vi "PID_TempControl.vi"() -> ()   [LabVIEW 2021]
uses:
  <vilib>/addons/control/pid/pid.llb/PID (DBL).vi
  <vilib>/addons/control/pid/NI_PID_pid.lvlib
panel:
  out "Meter":dbl(knob) scale=0.0..100.0
  in  "Dial":dbl(knob) scale=0.0..150.0
  in  "stop":bool
  out "Grafico de salidas":T1(graph)
  in  "PID gains":T2={"proportional gain (Kc)"=1.0, "integral time (Ti, min)"=0.01, "derivative time (Td, min)"=0.0} {"derivative time (Td, min)" format="%.3f"; "integral time (Ti, min)" format="%.3f"; "proportional gain (Kc)" format="%.3f"}
  out "Termometro":dbl(slide) scale=-2.0..150.0
  in  "Seleccionar temperatura (°c)":dbl(knob) scale=-2.0..150.0
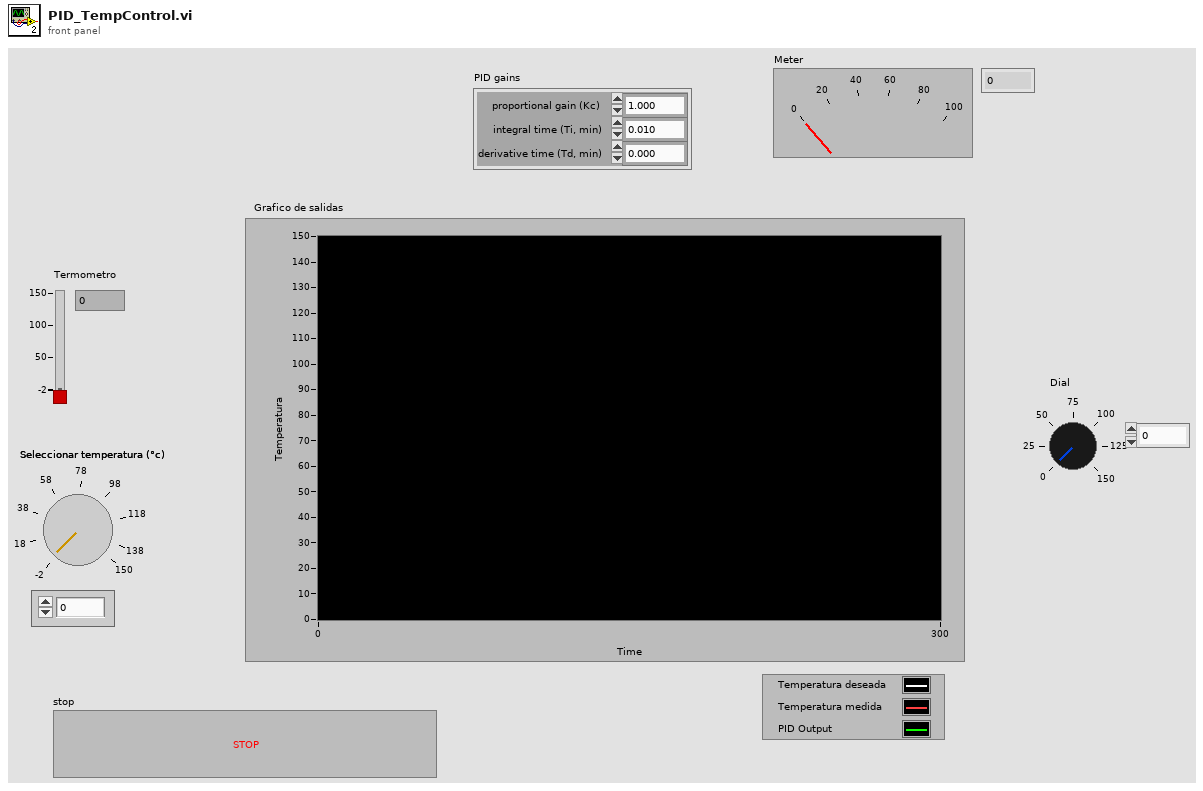
[diagram p1: front panel]
types:
  T1 = cluster{"Seleccionar temperatura (°c)":dbl, dbl, "output":dbl}
  T2 = cluster{"proportional gain (Kc)":dbl, "integral time (Ti, min)":dbl, "derivative time (Td, min)":dbl}
  T3 = cluster{"Seleccionar temperatura (°c)":dbl, "Dial":dbl, "output":dbl}
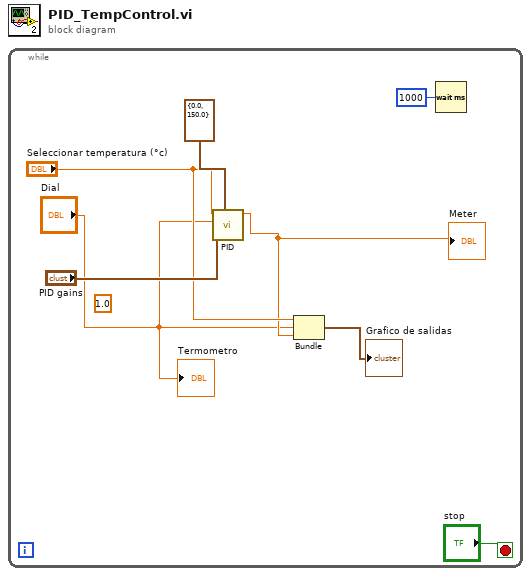
[diagram p0: block diagram]
diagram:
  n1 = while {
    stop <- "stop" stop-if-true
    (unwired) 1.0 ("y")
    n2 = call-poly <vilib>:"PID.vi"("output range"=cluster{"output low":dbl, "output high":dbl} {"output low"=0.0, "output high"=150.0}, "PID gains"="PID gains", "process variable"="Dial", "setpoint"="Seleccionar temperatura (°c)") -> ("output"=w2:dbl)  [unwired: 6 in, 1 out]
    "Meter" <- w2
    n3 = Bundle("Seleccionar temperatura (°c)"="Seleccionar temperatura (°c)", "Dial"="Dial", "output"=w2) -> (→"Grafico de salidas":T3)  [unwired: 1 in]
    n4 = Wait (ms)(milliseconds to wait=u32 1000) -> ()  [unwired: 1 out]
    "Termometro" <- "Dial"
  }
